vi "Write Pin.vi"(0 "NXP in":refnum<class "NXP.lvclass">, 5 "VISA resource name":refnum<visa-resource-name>, 7 "Pin":dbl, 9 "1/0":bool, 11 "error in (no error)":errorcluster) -> (4 "NXP out":refnum<class "NXP.lvclass">, 6 "VISA resource name 2":refnum<visa-resource-name>, 10 "Read":string, 15 "error out":errorcluster)   [LabVIEW 2020, in "NXP.lvclass"]
uses:
  NXP.lvclass
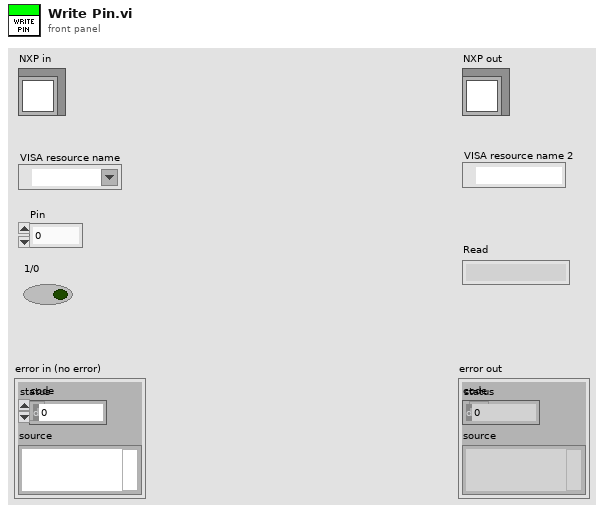
[diagram p1: front panel]
types:
  T1 = enum16{"Write", "Read", "Config", "Reset", "Close"}
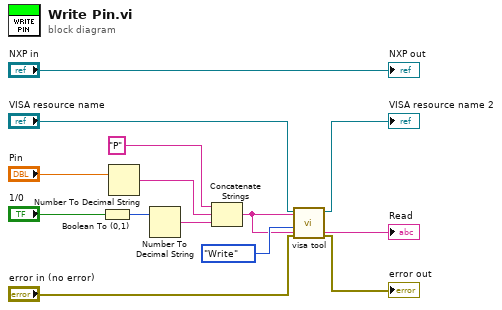
[diagram p0: block diagram]
diagram:
  n1 = Boolean To (0,1)(Boolean="1/0") -> (0, 1=w12:i16)
  n2 = Number To Decimal String(number="Pin") -> (decimal integer string=w9:string)  [unwired: 1 in]
  n3 = Number To Decimal String(number=w12) -> (decimal integer string=w10:string)  [unwired: 1 in]
  n4 = Concatenate Strings("P" ("string"), w9, w10) -> (w3:string)
  "Read" <- w3
  n5 = call "visa tool.vi"("error in (no error)"="error in (no error)", "Opciones"=T1."Write", "Write"=w3, "VISA com port"="VISA resource name") -> ("error out"=→"error out":errorcluster, "VISA com port 2"=→"VISA resource name 2":refnum<visa-resource-name>)  [unwired: 5 in, 1 out]
  "NXP out" <- "NXP in"
